vi "Operator.vi"() -> ()   [LabVIEW 2019]
uses:
  <vilib>/Rock Robotics/WPI/ThirdParty/Phoenix-LabVIEW/Motor Controller/Controls/CTRE_Phoenix_MotorControl_ControlMode.ctl
  <vilib>/Rock Robotics/WPI/Solenoid/WPI_SolenoidValue.ctl
  <vilib>/Rock Robotics/WPI/Utilities/WPI_GetSetVariantRefNum.vi
  <vilib>/Rock Robotics/WPI/Solenoid/WPI_SolenoidSetEnum.vi
  <vilib>/Rock Robotics/Network Tables/NT Write Boolean Array.vi
  <vilib>/Rock Robotics/Network Tables/NT Write Numeric Array.vi
panel:
  in  "Intake":T1 items=["PercentOutput"=0, "Position"=1, "Velocity"=2, "Current"=3, "Follower"=5, "MotionProfile"=6, "MotionMagic"=7, "MotionProfileArc"=10, "Disabled"=15]
  in  "Intake":T1 items=["PercentOutput"=0, "Position"=1, "Velocity"=2, "Current"=3, "Follower"=5, "MotionProfile"=6, "MotionMagic"=7, "MotionProfileArc"=10, "Disabled"=15]
  in  "Control Panel 2":T1 items=["PercentOutput"=0, "Position"=1, "Velocity"=2, "Current"=3, "Follower"=5, "MotionProfile"=6, "MotionMagic"=7, "MotionProfileArc"=10, "Disabled"=15]
  in  "Control Panel":T1 items=["PercentOutput"=0, "Position"=1, "Velocity"=2, "Current"=3, "Follower"=5, "MotionProfile"=6, "MotionMagic"=7, "MotionProfileArc"=10, "Disabled"=15]
  in  "Winch 4":T1 items=["PercentOutput"=0, "Position"=1, "Velocity"=2, "Current"=3, "Follower"=5, "MotionProfile"=6, "MotionMagic"=7, "MotionProfileArc"=10, "Disabled"=15]
  in  "Winch 3":T1 items=["PercentOutput"=0, "Position"=1, "Velocity"=2, "Current"=3, "Follower"=5, "MotionProfile"=6, "MotionMagic"=7, "MotionProfileArc"=10, "Disabled"=15]
  in  "Climber 2":T1 items=["PercentOutput"=0, "Position"=1, "Velocity"=2, "Current"=3, "Follower"=5, "MotionProfile"=6, "MotionMagic"=7, "MotionProfileArc"=10, "Disabled"=15]
  in  "Climber":T1 items=["PercentOutput"=0, "Position"=1, "Velocity"=2, "Current"=3, "Follower"=5, "MotionProfile"=6, "MotionMagic"=7, "MotionProfileArc"=10, "Disabled"=15]
  in  "Output":T1 items=["PercentOutput"=0, "Position"=1, "Velocity"=2, "Current"=3, "Follower"=5, "MotionProfile"=6, "MotionMagic"=7, "MotionProfileArc"=10, "Disabled"=15]
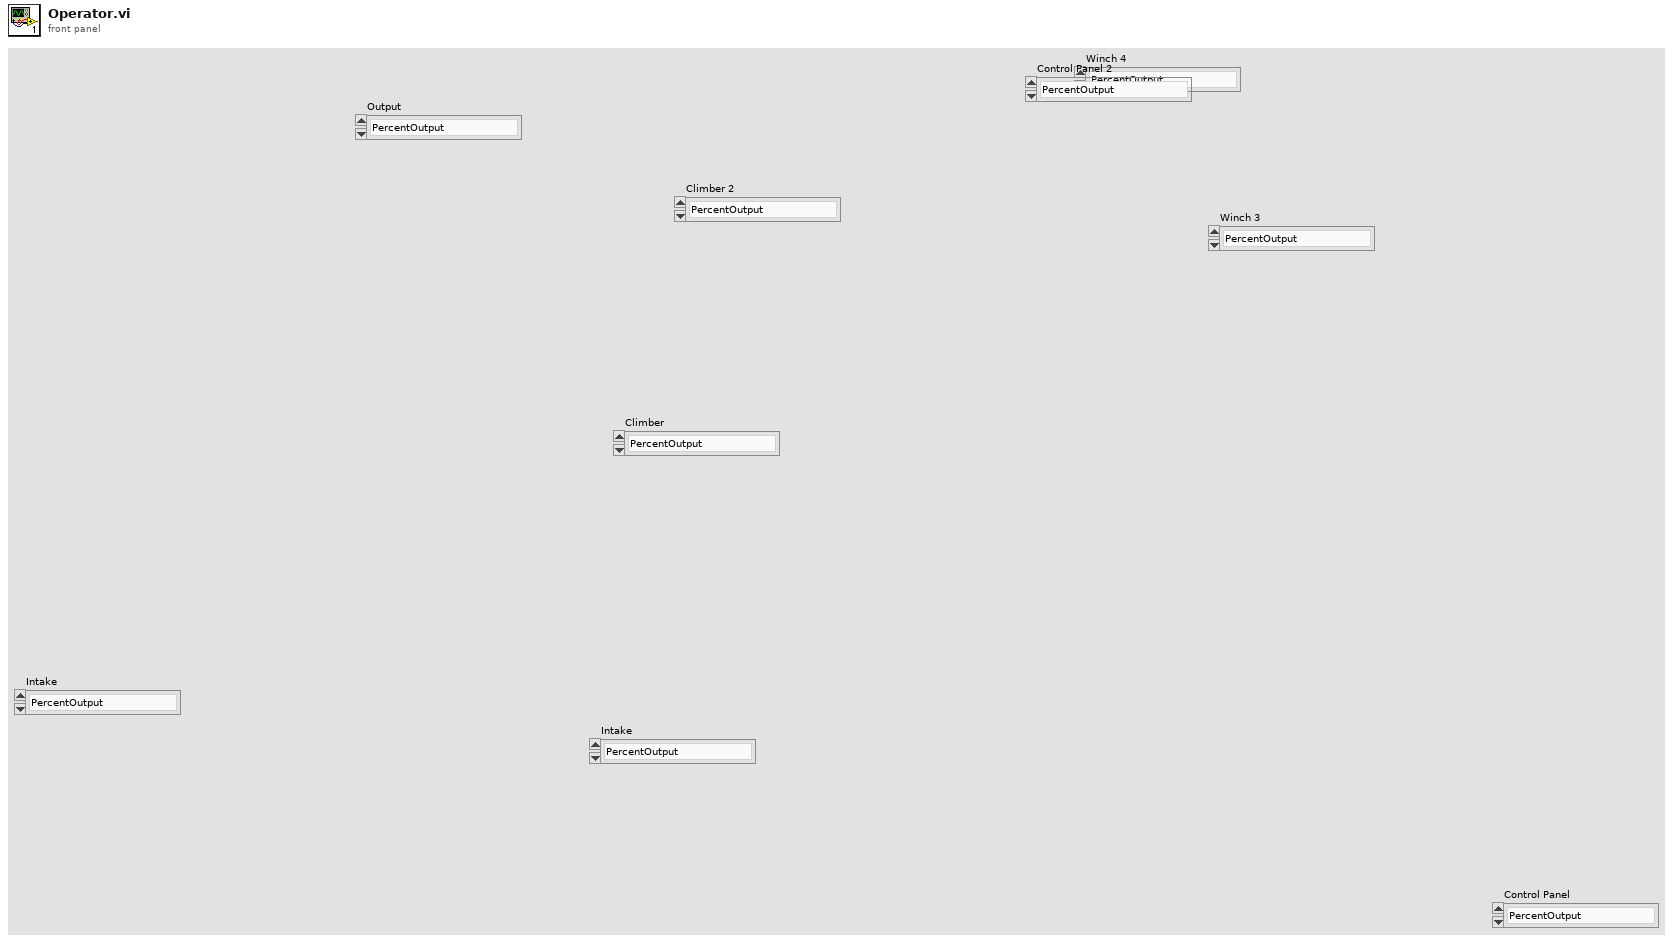
[diagram p1: front panel]
types:
  T1 = typedef "CTRE_Phoenix_MotorControl_ControlMode.ctl" = u16
  T2 = typedef "WPI_JoystickDevRef.ctl" = cluster{"Device":T3}
  T3 = typedef "WPI_JoystickDeviceEnum.ctl" = enum16{"USB 0", "USB 1", "USB 2", "USB 3", "USB 4", "USB 5"}
  T4 = typedef "WPI_MotorControlDeviceRef.ctl" = cluster{"DeviceStatus":errorcluster, "Type":T5, "PWM":cluster{"PWM Channel":T6, "DeadBand":T7}, "CAN":cluster{"Device Number":u8, "SetOutput VI Ref":variant, "GetOutput VI Ref":variant, "Enable VI Ref":variant, "Disable VI Ref":variant, "Data":variant}, "Invert":bool, "DIO PWM":cluster{"PWM \"Enable\" Channel":T6, "DIOChannel":T8, "PWM Rate":dbl}}
  T5 = typedef "WPI_MotorControlType.ctl" = enum16{"PWM", "CAN", "DIO PWM"}
  T6 = typedef "FPGA_DIOPWMChannel.ctl" = enum8{"PWM 0", "PWM 1", "PWM 2", "PWM 3", "PWM 4", "PWM 5", "PWM 6", "PWM 7", "PWM 8", "PWM 9", "PWM MXP 0", "PWM MXP 1", "PWM MXP 2", "PWM MXP 3", "PWM MXP 4", "PWM MXP 5", "PWM MXP 6", "PWM MXP 7", "PWM MXP 8", "PWM MXP 9", "Invalid"}
  T7 = typedef "WPI_PWMDeadband.ctl" = cluster{"Name":string, "maxPositivePwm":i32, "minPositivePwm":i32, "centerPwm":i32, "maxNegativePwm":i32, "minNegativePwm":i32, "angularRange":u16}
  T8 = typedef "FPGA_DIOChannel.ctl" = enum8{"DIO 0", "DIO 1", "DIO 2", "DIO 3", "DIO 4", "DIO 5", "DIO 6", "DIO 7", "DIO 8", "DIO 9", "DIO MXP 0", "DIO MXP 1", "DIO MXP 2", "DIO MXP 3", "DIO MXP 4", "DIO MXP 5", "DIO MXP 6", "DIO MXP 7", "DIO MXP 8", "DIO MXP 9", "DIO MXP 10", "DIO MXP 11", "DIO MXP 12", "DIO MXP 13", "DIO MXP 14", "DIO MXP 15", "SPI Port CS1", "SPI Port CS2", "SPI Port CS3", "SPI Port MISO", "SPI Port MOSI", "Invalid"}
  T9 = typedef "WPI_SolenoidValue.ctl" = enum16{"Off", "On", "Forward", "Reverse"}
  T10 = typedef "WPI_SolenoidDevRef.ctl" = cluster{"DevStatus":errorcluster, "Pneumatics Control Module":u8, "Forward Solenoid Channel":T11, "Reverse Solenoid Channel":T11}
  T11 = typedef "WPI_SolenoidChannel.ctl" = enum8{"Solenoid 0", "Solenoid 1", "Solenoid 2", "Solenoid 3", "Solenoid 4", "Solenoid 5", "Solenoid 6", "Solenoid 7", "Invalid"}
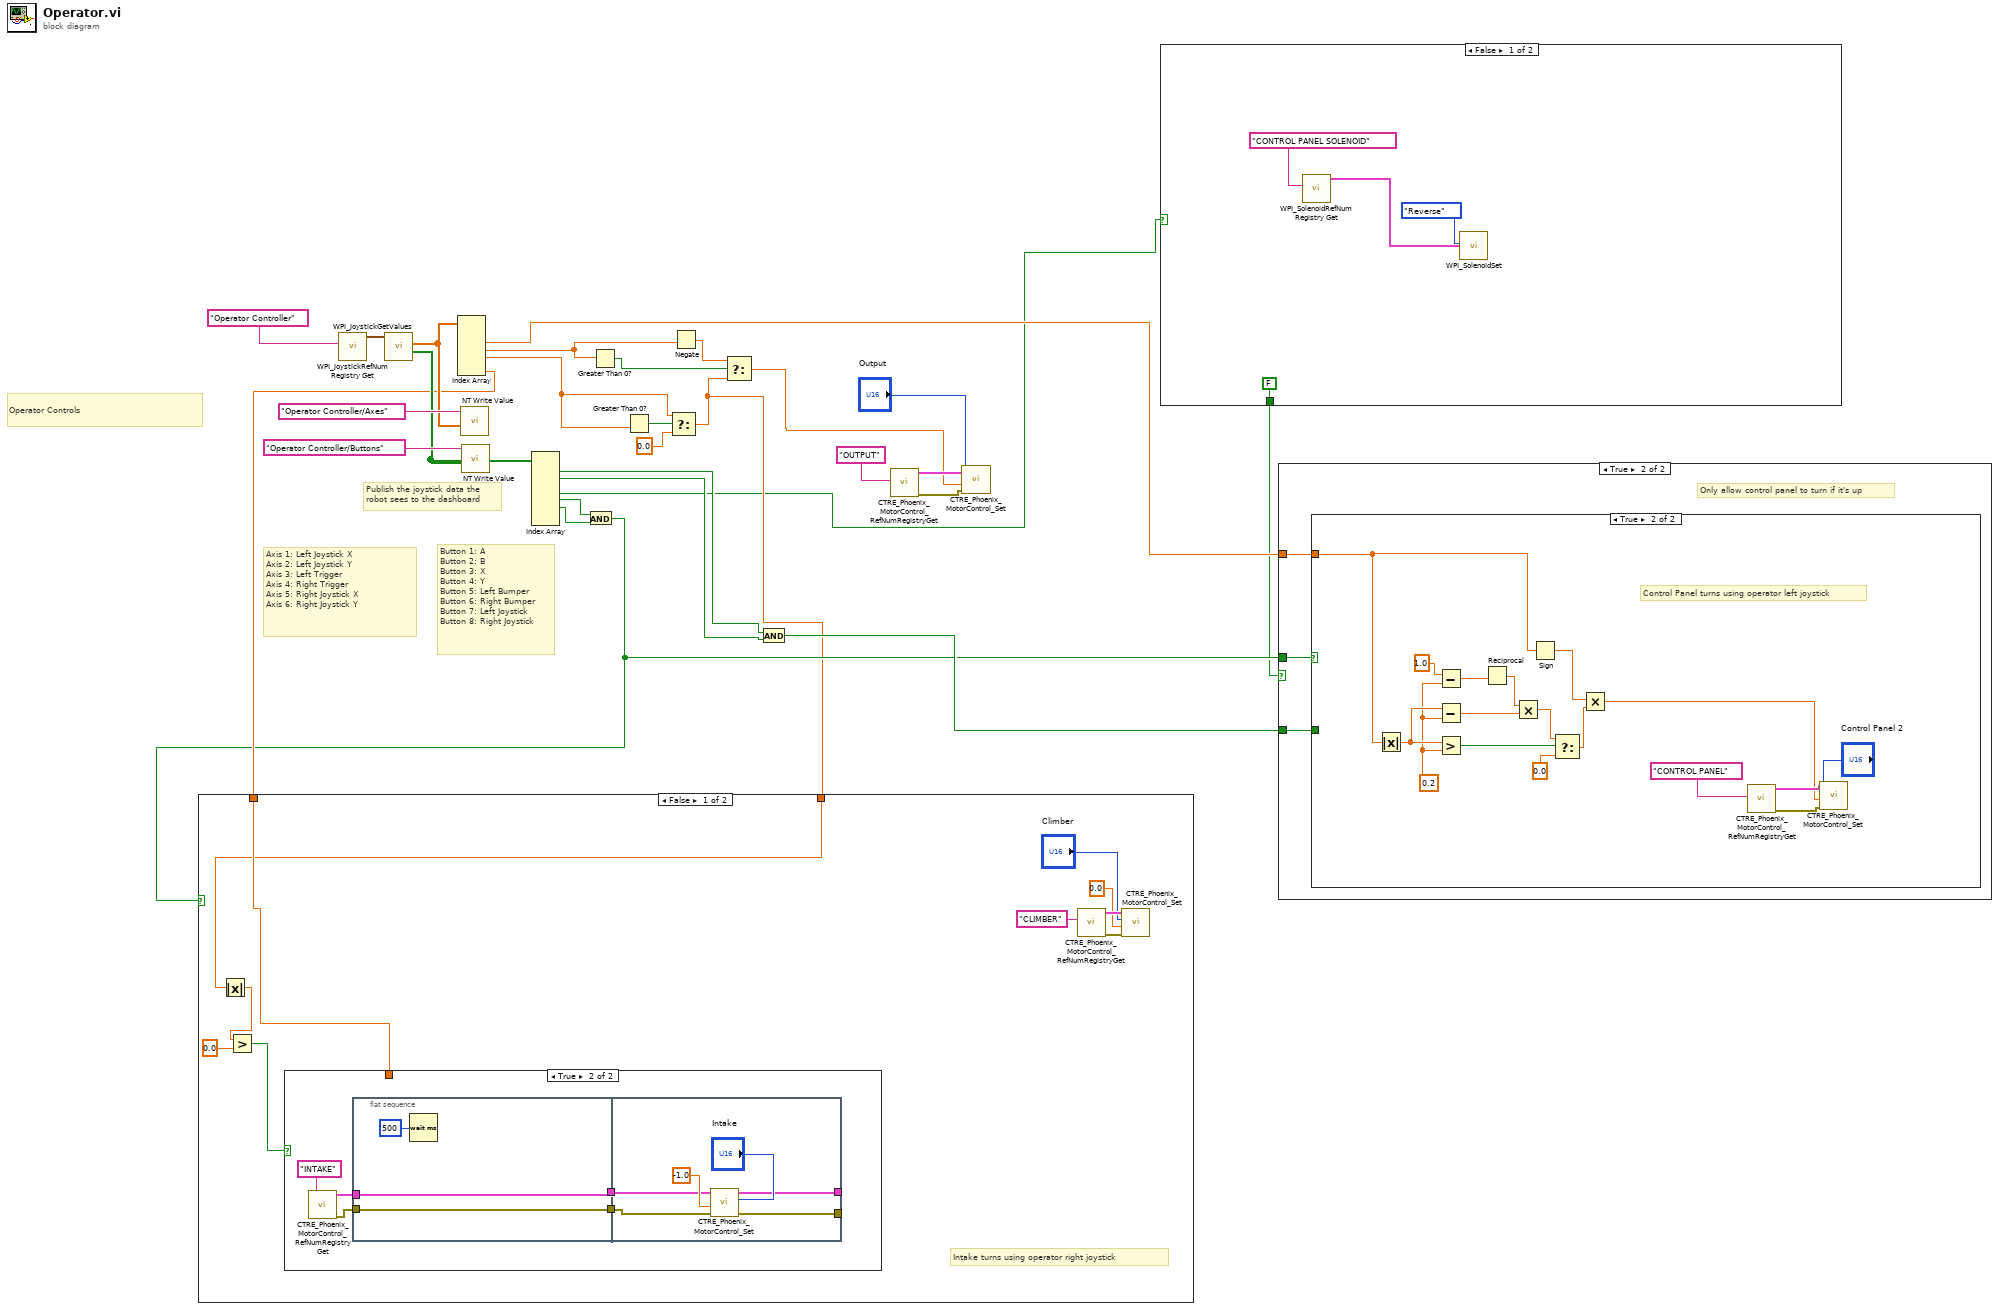
[diagram p0: block diagram]
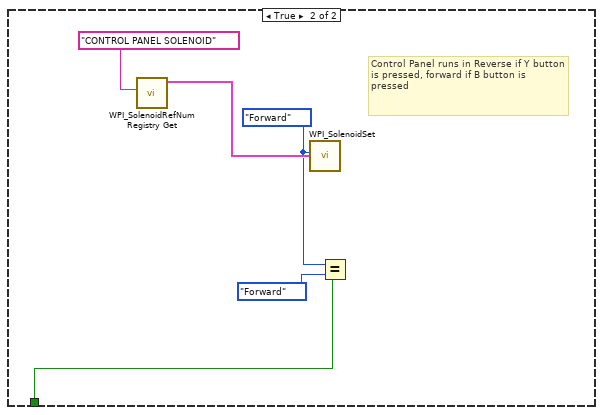
[diagram p2: hidden frame]
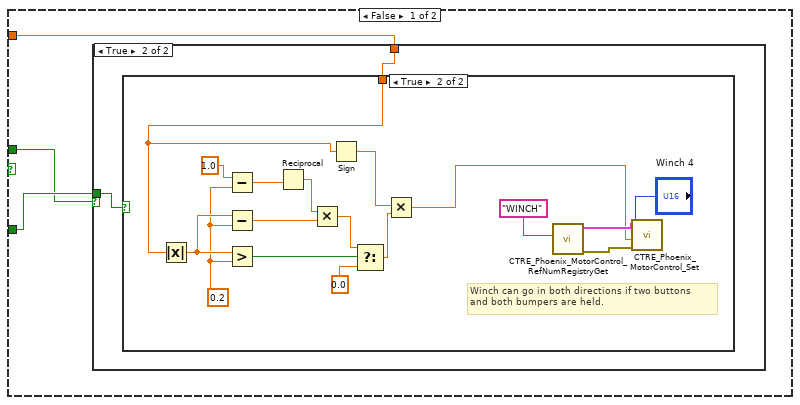
[diagram p3: hidden frame]
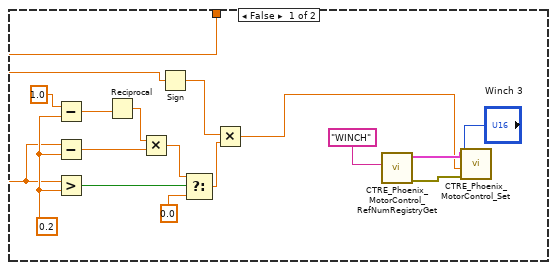
[diagram p5: hidden frame]
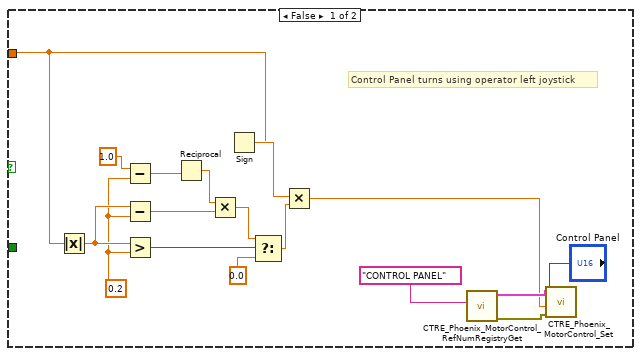
[diagram p6: hidden frame]
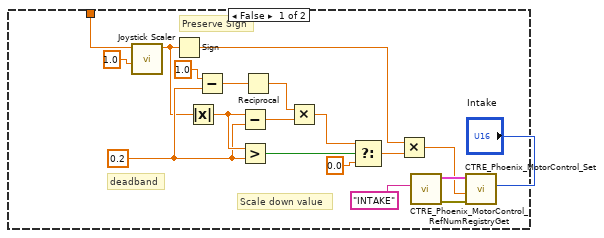
[diagram p7: hidden frame]
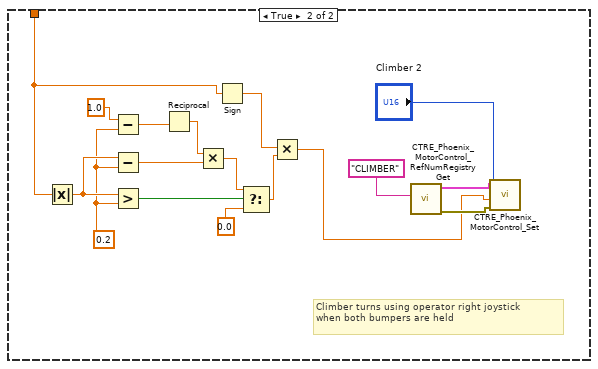
[diagram p8: hidden frame]
diagram:
  # "Button 1: A\nButton 2: B\nButton 3: X\nButton 4: Y\nButton 5: Left Bumper\nButton 6: Right Bumper\nButton 7: Left Joystick\nButton 8: Right Joystick"
  # "Axis 1: Left Joystick X\nAxis 2: Left Joystick Y\nAxis 3: Left Trigger\nAxis 4: Right Trigger\nAxis 5: Right Joystick X\nAxis 6: Right Joystick Y"
  # "Operator Controls"
  # "Publish the joystick data the\nrobot sees to the dashboard"
  n1 = call <vilib>:"WPI_JoystickRefNum Registry Get.vi"("refnum name"="Operator Controller") -> ("JoystickDevRef"=w23:T2)  [unwired: 1 in, 9 out]
  n2 = call <vilib>:"WPI_JoystickGetValues.vi"("JoystickDevRef"=w23) -> ("Buttons"=w19:bool[], "Axes"=w20:dbl[])  [unwired: 6 in, 3 out]
  n3 = Index Array(array=w20) -> (element #2=w9:dbl, element #3=w14:dbl, element #4=w15:dbl, element #6=w13:dbl)  [unwired: 6 in, 2 out]
  n4 = call-poly <vilib>:"NT Write Value.vi"("Numeric Array"=w20, "Name"="Operator Controller/Axes") -> ()  [unwired: 9 in, 1 out]
  n5 = call-poly <vilib>:"NT Write Value.vi"("Boolean Array"=w19, "Name"="Operator Controller/Buttons") -> ()  [unwired: 9 in, 1 out]
  n6 = Index Array(array=w19) -> (element #1=w8:bool, element #2=w4:bool, element #4=w1:bool, element #5=w12:bool, element #6=w11:bool)  [unwired: 8 in, 3 out]
  n7 = And(x=w12, y=w11) -> (x .and. y?=w6:bool)
  n8 = Greater Than 0?(x=w14) -> (x > 0?=w18:bool)
  n9 = Greater Than 0?(x=w15) -> (x > 0?=w17:bool)
  n10 = Select(t=w15, s=w17, f=0.0) -> (s? t:f=w3:dbl)
  n11 = case shown="False" w6 {
    tunnel: w13 -> [w30 w72]
    tunnel: w3 -> [w29 _]
    frame False {
      # "Intake turns using operator right joystick"
      n12 = Absolute Value(x=w29) -> (abs(x)=w32:dbl)
      n13 = Greater?(x=w32, y=0.0) -> (0:w31:bool)
      n14 = case shown="True" w31 {
        tunnel: w30 -> [w39 _]
        frame False {
          w44 = 0.2 ("y")
          # "Preserve Sign"
          # "deadband"
          # "Scale down value"
          n15 = call "Joystick Scaler.vi"("Scaler"=1.0, "Joystick Value"=w39) -> ("Final Joystick Value"=w41:dbl)  [unwired: 9 in]
          n16 = Sign(1:w41) -> (0:w40:dbl)
          n17 = Absolute Value(x=w41) -> (abs(x)=w45:dbl)
          n18 = Subtract(x=1.0, y=w44) -> (x-y=w47:dbl)
          n19 = Subtract(x=w45, y=w44) -> (x-y=w43:dbl)
          n20 = Greater?(x=w45, y=w44) -> (0:w52:bool)
          n21 = Reciprocal(x=w47) -> (1/x=w46:dbl)
          n22 = Multiply(x=w46, y=w43) -> (x*y=w49:dbl)
          n23 = Select(t=w49, s=w52, f=0.0) -> (s? t:f=w50:dbl)
          n24 = Multiply(x=w40, y=w50) -> (x*y=w42:dbl)
          n25 = call <vilib>:"CTRE_Phoenix_MotorControl_RefNumRegistryGet.vi"("refnum name"="INTAKE") -> ("error out"=w56:errorcluster, "PhoenixMotorControlDevRef"=w55:T4)  [unwired: 9 in]
          n26 = call <vilib>:"CTRE_Phoenix_MotorControl_Set.vi"("error in (no error)"=w56, "Output"=w42, "Control Mode"="Intake", "PhoenixMotorControlDevRef"=w55) -> ()  [unwired: 6 in, 2 out]
        }
        frame True {
          n27 = call <vilib>:"CTRE_Phoenix_MotorControl_RefNumRegistryGet.vi"("refnum name"="INTAKE") -> ("error out"=w59:errorcluster, "PhoenixMotorControlDevRef"=w61:T4)  [unwired: 9 in]
          n28 = flat-sequence {
            tunnel: [w65] -> w62
            tunnel: w61 -> [w65]
            tunnel: [w64] -> w60
            tunnel: w59 -> [w64]
            tunnel: w62 -> [w69]
            tunnel: w60 -> [w68]
            tunnel: [w67] -> _
            tunnel: [w66] -> _
            frame #0 {
              n29 = Wait (ms)(milliseconds to wait=u32 500) -> ()  [unwired: 1 out]
            }
            frame #1 {
              n30 = call <vilib>:"CTRE_Phoenix_MotorControl_Set.vi"("error in (no error)"=w68, "Output"=-1.0, "Control Mode"="Intake", "PhoenixMotorControlDevRef"=w69) -> ("error out"=w66:errorcluster, "PhoenixMotorControlDevRef"=w67:T4)  [unwired: 6 in]
            }
          }
        }
      }
      n31 = call <vilib>:"CTRE_Phoenix_MotorControl_RefNumRegistryGet.vi"("refnum name"="CLIMBER") -> ("error out"=w36:errorcluster, "PhoenixMotorControlDevRef"=w37:T4)  [unwired: 9 in]
      n32 = call <vilib>:"CTRE_Phoenix_MotorControl_Set.vi"("error in (no error)"=w36, "Output"=0.0, "Control Mode"="Climber", "PhoenixMotorControlDevRef"=w37) -> ()  [unwired: 6 in, 2 out]
    }
    frame True {
      w76 = 0.2 ("y")
      # "Climber turns using operator right joystick\nwhen both bumpers are held"
      n33 = Absolute Value(x=w72) -> (abs(x)=w77:dbl)
      n34 = Subtract(x=1.0, y=w76) -> (x-y=w79:dbl)
      n35 = Subtract(x=w77, y=w76) -> (x-y=w75:dbl)
      n36 = Greater?(x=w77, y=w76) -> (0:w84:bool)
      n37 = Reciprocal(x=w79) -> (1/x=w78:dbl)
      n38 = Multiply(x=w78, y=w75) -> (x*y=w81:dbl)
      n39 = Sign(1:w72) -> (0:w74:dbl)
      n40 = Select(t=w81, s=w84, f=0.0) -> (s? t:f=w82:dbl)
      n41 = Multiply(x=w74, y=w82) -> (x*y=w73:dbl)
      n42 = call <vilib>:"CTRE_Phoenix_MotorControl_RefNumRegistryGet.vi"("refnum name"="CLIMBER") -> ("error out"=w86:errorcluster, "PhoenixMotorControlDevRef"=w87:T4)  [unwired: 9 in]
      n43 = call <vilib>:"CTRE_Phoenix_MotorControl_Set.vi"("error in (no error)"=w86, "Output"=w73, "Control Mode"="Climber 2", "PhoenixMotorControlDevRef"=w87) -> ()  [unwired: 6 in, 2 out]
    }
  }
  n44 = Negate(x=w14) -> (-x=w2:dbl)
  n45 = Select(t=w2, s=w18, f=w3) -> (s? t:f=w10:dbl)
  n46 = And(x=w8, y=w4) -> (x .and. y?=w7:bool)
  n47 = call <vilib>:"CTRE_Phoenix_MotorControl_RefNumRegistryGet.vi"("refnum name"="OUTPUT") -> ("error out"=w26:errorcluster, "PhoenixMotorControlDevRef"=w27:T4)  [unwired: 9 in]
  n48 = call <vilib>:"CTRE_Phoenix_MotorControl_Set.vi"("error in (no error)"=w26, "Output"=w10, "Control Mode"="Output", "PhoenixMotorControlDevRef"=w27) -> ()  [unwired: 6 in, 2 out]
  n49 = case shown="False" w1 {
    tunnel: [FALSE w93] -> w5
    frame False {
      n50 = call <vilib>:"WPI_SolenoidRefNum Registry Get.vi"("refnum name"="CONTROL PANEL SOLENOID") -> ("SolenoidDevRef"=w91:T10)  [unwired: 9 in, 1 out]
      n51 = call-poly <vilib>:"WPI_SolenoidSet.vi"("Value"=WPI_SolenoidValue."Reverse", "SolenoidDevRef"=w91) -> ()  [unwired: 8 in, 2 out]
    }
    frame True {
      w95 = WPI_SolenoidValue."Forward" ("Value")
      # "Control Panel runs in Reverse if Y button is pressed, forward if B button is pressed"
      n52 = call <vilib>:"WPI_SolenoidRefNum Registry Get.vi"("refnum name"="CONTROL PANEL SOLENOID") -> ("SolenoidDevRef"=w96:T10)  [unwired: 9 in, 1 out]
      n53 = call-poly <vilib>:"WPI_SolenoidSet.vi"("Value"=w95, "SolenoidDevRef"=w96) -> ()  [unwired: 8 in, 2 out]
      n54 = Equal?(x=w95, y=WPI_SolenoidValue."Forward") -> (x = y?=w93:bool)
    }
  }
  n55 = case shown="True" w5 {
    tunnel: w9 -> [w99 w138]
    tunnel: w7 -> [w100 w137]
    tunnel: w6 -> [w98 w136]
    frame False {
      n56 = case shown="True" w98 {
        tunnel: w100 -> [_ w102]
        tunnel: w99 -> [_ w101]
        frame False {
        }
        frame True {
          n57 = case shown="True" w102 {
            tunnel: w101 -> [w103 w119]
            frame False {
              w107 = 0.2 ("y")
              n58 = Subtract(x=1.0, y=w107) -> (x-y=w109:dbl)
              n59 = Subtract(x=w103, y=w107) -> (x-y=w106:dbl)
              n60 = Greater?(x=w103, y=w107) -> (0:w114:bool)
              n61 = Reciprocal(x=w109) -> (1/x=w108:dbl)
              n62 = Multiply(x=w108, y=w106) -> (x*y=w111:dbl)
              n63 = Sign(1:w103) -> (0:w105:dbl)
              n64 = Select(t=w111, s=w114, f=0.0) -> (s? t:f=w112:dbl)
              n65 = Multiply(x=w105, y=w112) -> (x*y=w104:dbl)
              n66 = call <vilib>:"CTRE_Phoenix_MotorControl_RefNumRegistryGet.vi"("refnum name"="WINCH") -> ("error out"=w117:errorcluster, "PhoenixMotorControlDevRef"=w116:T4)  [unwired: 9 in]
              n67 = call <vilib>:"CTRE_Phoenix_MotorControl_Set.vi"("error in (no error)"=w117, "Output"=w104, "Control Mode"="Winch 3", "PhoenixMotorControlDevRef"=w116) -> ()  [unwired: 6 in, 2 out]
            }
            frame True {
              w123 = 0.2 ("y")
              # "Winch can go in both directions if two buttons\nand both bumpers are held."
              n68 = Absolute Value(x=w119) -> (abs(x)=w124:dbl)
              n69 = Subtract(x=1.0, y=w123) -> (x-y=w126:dbl)
              n70 = Subtract(x=w124, y=w123) -> (x-y=w122:dbl)
              n71 = Greater?(x=w124, y=w123) -> (0:w131:bool)
              n72 = Reciprocal(x=w126) -> (1/x=w125:dbl)
              n73 = Multiply(x=w125, y=w122) -> (x*y=w128:dbl)
              n74 = Sign(1:w119) -> (0:w121:dbl)
              n75 = Select(t=w128, s=w131, f=0.0) -> (s? t:f=w129:dbl)
              n76 = Multiply(x=w121, y=w129) -> (x*y=w120:dbl)
              n77 = call <vilib>:"CTRE_Phoenix_MotorControl_RefNumRegistryGet.vi"("refnum name"="WINCH") -> ("error out"=w134:errorcluster, "PhoenixMotorControlDevRef"=w133:T4)  [unwired: 9 in]
              n78 = call <vilib>:"CTRE_Phoenix_MotorControl_Set.vi"("error in (no error)"=w134, "Output"=w120, "Control Mode"="Winch 4", "PhoenixMotorControlDevRef"=w133) -> ()  [unwired: 6 in, 2 out]
            }
          }
        }
      }
    }
    frame True {
      # "Only allow control panel to turn if it's up"
      n79 = case shown="True" w136 {
        tunnel: w138 -> [w140 w156]
        tunnel: w137 -> [_ _]
        frame False {
          w143 = 0.2 ("y")
          # "Control Panel turns using operator left joystick"
          n80 = Absolute Value(x=w140) -> (abs(x)=w144:dbl)
          n81 = Subtract(x=1.0, y=w143) -> (x-y=w146:dbl)
          n82 = Subtract(x=w144, y=w143) -> (x-y=w142:dbl)
          n83 = Greater?(x=w144, y=w143) -> (0:w151:bool)
          n84 = Reciprocal(x=w146) -> (1/x=w145:dbl)
          n85 = Multiply(x=w145, y=w142) -> (x*y=w148:dbl)
          n86 = Sign(1:w140) -> (0:w141:dbl)
          n87 = Select(t=w148, s=w151, f=0.0) -> (s? t:f=w149:dbl)
          n88 = Multiply(x=w141, y=w149) -> (x*y=w139:dbl)
          n89 = call <vilib>:"CTRE_Phoenix_MotorControl_RefNumRegistryGet.vi"("refnum name"="CONTROL PANEL") -> ("error out"=w154:errorcluster, "PhoenixMotorControlDevRef"=w153:T4)  [unwired: 9 in]
          n90 = call <vilib>:"CTRE_Phoenix_MotorControl_Set.vi"("error in (no error)"=w154, "Output"=w139, "Control Mode"="Control Panel", "PhoenixMotorControlDevRef"=w153) -> ()  [unwired: 6 in, 2 out]
        }
        frame True {
          w160 = 0.2 ("y")
          # "Control Panel turns using operator left joystick"
          n91 = Absolute Value(x=w156) -> (abs(x)=w161:dbl)
          n92 = Subtract(x=1.0, y=w160) -> (x-y=w163:dbl)
          n93 = Subtract(x=w161, y=w160) -> (x-y=w159:dbl)
          n94 = Greater?(x=w161, y=w160) -> (0:w168:bool)
          n95 = Reciprocal(x=w163) -> (1/x=w162:dbl)
          n96 = Multiply(x=w162, y=w159) -> (x*y=w165:dbl)
          n97 = Sign(1:w156) -> (0:w158:dbl)
          n98 = Select(t=w165, s=w168, f=0.0) -> (s? t:f=w166:dbl)
          n99 = Multiply(x=w158, y=w166) -> (x*y=w157:dbl)
          n100 = call <vilib>:"CTRE_Phoenix_MotorControl_RefNumRegistryGet.vi"("refnum name"="CONTROL PANEL") -> ("error out"=w171:errorcluster, "PhoenixMotorControlDevRef"=w170:T4)  [unwired: 9 in]
          n101 = call <vilib>:"CTRE_Phoenix_MotorControl_Set.vi"("error in (no error)"=w171, "Output"=w157, "Control Mode"="Control Panel 2", "PhoenixMotorControlDevRef"=w170) -> ()  [unwired: 6 in, 2 out]
        }
      }
    }
  }
